vi "Append Pass Result.vi"(7 "Description":string, 8 "error in (no error)":errorcluster, 9 "Data":T1, 10 "Result Type":T2, 11 "LUnit Test Case In":refnum<class "LUnit Test Case.lvclass">) -> (0 "error out":errorcluster, 3 "LUnit Test Case Out":refnum<class "LUnit Test Case.lvclass">)   [LabVIEW 2020, in "LUnit Test Case.lvclass"]
doc: "Generates a pass result for the calling test method. A description and message may be provided."
uses:
  LUnit Test Case.lvclass
  Result/Type.ctl
  Result/Result.ctl
  Result/Status.ctl
  LUnit Test Case.lvclass/LUnit Test Case.ctl
  <vilib>/Utility/error.llb/Clear Errors.vi
  Result/Result.lvlib
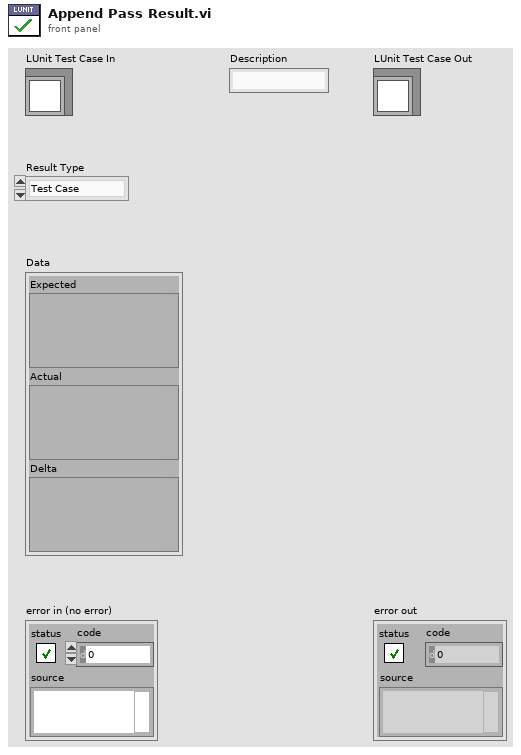
[diagram p1: front panel]
types:
  T1 = cluster{"Expected":variant, "Actual":variant, "Delta":variant}
  T2 = typedef "Result.lvlib/Type.ctl" = enum16{"Test Case", "Test Suite", "Test Run", "Pass", "Fail", "Skip", "Pass if", "Fail if", "Pass if Error", "Fail if Error", "Pass if Equal", "Fail if Equal"}
  T3 = typedef "Result.lvlib/Result.ctl" = cluster{"Name":string, "Description":string, "Status":T4, "Result Type":T2, "Execution Time":dbl, "Data":cluster{"Expected":variant, "Actual":variant, "Delta":variant}}
  T4 = typedef "Result.lvlib/Status.ctl" = enum16{"", "Passed", "Failed", "Error", "Skipped", "Setup Error", "Broken", "Teardown Error"}
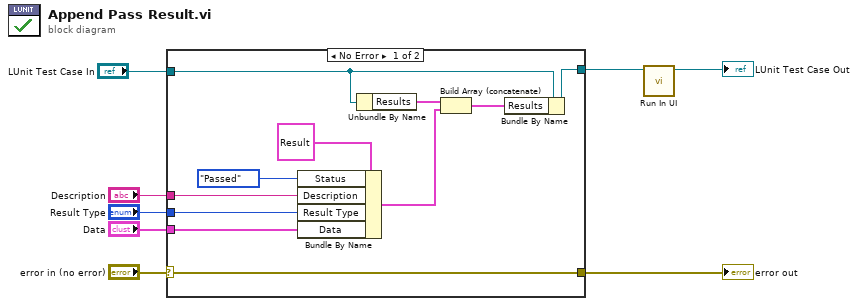
[diagram p0: block diagram]
diagram:
  n1 = case shown="No Error" "error in (no error)" {
    selector: "error in (no error)" -> [w18 w20]
    tunnel: "LUnit Test Case In" -> [w19 w21]
    tunnel: [w18 w20] -> w6
    tunnel: "Description" -> [w17 _]
    tunnel: [w16 w21] -> w4
    tunnel: "Result Type" -> [w14 _]
    tunnel: "Data" -> [w10 _]
    frame No Error {
      n2 = Bundle By Name(cluster=T3 {"Name"="", "Description"="", "Status"=enum."Passed", "Result Type"=enum."Pass", "Execution Time"=0.0, "Data"={"Expected"=variant, "Actual"=variant, "Delta"=variant}} ("Temporary Assertion Result"), "Status"=Status."Passed", "Description"=w17, "Result Type"=w14, "Data"=w10) -> (w15:T3)
      n3 = Unbundle By Name(w19) -> ("Results"=w13:T3[])
      n4 = Build Array (concatenate)(w13, w15) -> (w12:T3[])
      n5 = Bundle By Name(cluster=w19, "Results"=w12) -> (w16:refnum<class "LUnit Test Case.lvclass">)
    }
    frame Error {
    }
  }
  "error out" <- w6
  n6 = call "Run In UI.vi"("LUnit Test Case in"=w4) -> ("LUnit Test Case out"=→"LUnit Test Case Out":refnum<class "LUnit Test Case.lvclass">)  [unwired: 10 in]
